vi "Drive_Teleop.vi"(1 "Joystick_Out":T1={"Pilot Left Joystick X"=0.007874015748031496, "Pilot Left Joystick Y"=-0.0, "Pilot A Button"=FALSE, "Pilot B Button"=FALSE, "Pilot X Button"=FALSE, "Pilot Y Button"=FALSE, "Pilot Left Bumper"=FALSE, "Pilot Right Bumper"=FALSE, "Pilot View Button"=FALSE, "Pilot Menu Button"=FALSE, "Pilot Left Joystick Press"=FALSE, "Pilot Right Joystick Press"=FALSE, "Pilot Left Trigger"=0.0, "Pilot Right Joystick X"=0.0, "Pilot Right Joystick Y"=0.0, "Pilot Right Trigger"=0.0, "Copilot Left Joystick X"=0.05511811023622047, "Copilot Left Joystick Y"=0.023622047244094488, "Copilot A Button"=FALSE, "Copilot B Button"=FALSE, "Copilot X Button"=FALSE, "Copilot Y Button"=FALSE, "Copilot Left Bumper"=FALSE, "Copilot Right Bumper"=FALSE, "Copilot View Button"=FALSE, "Copilot Menu Button"=FALSE, "Copilot Left Joystick Press"=FALSE, "Copilot Right Joystick Press"=FALSE, "Copilot Left Trigger"=0.0, "Copilot Right Joystick X"=-0.015748031496062992, "Copilot Right Joystick Y"=0.05511811023622047, "Copilot Right Trigger"=0.0, "Pilot D-pad North"=FALSE, "Pilot D-pad South"=FALSE, "Pilot D-pad East"=FALSE, "Pilot D-pad West"=FALSE, "Pilot D-pad NE "=FALSE, "Pilot D-pad SE"=FALSE, "Pilot D-pad SW"=FALSE, "Pilot D-pad NW"=FALSE, "CoPilot D-pad North"=FALSE, "CoPilot D-pad South"=FALSE, "CoPilot D-pad East"=FALSE, "CoPilot D-pad West"=FALSE, "CoPilot D-pad NE"=FALSE, "CoPilot D-pad SE"=FALSE, "CoPilot D-pad SW"=FALSE, "CoPilot D-pad NW"=FALSE, "Pilot Left Trigger Pressed"=FALSE, "Pilot Right Trigger Pressed"=FALSE, "CoPilot Left Trigger Pressed"=FALSE, "CoPilot Right Trigger Pressed"=FALSE}) -> ()   [LabVIEW 2020]
uses:
  Utility VIs/Joystick_Controls.ctl
  Subsystems/Drive/Drive_Cluster.ctl
  Subsystems/Drive/Drive_Control_States.ctl
  Subsystems/Drive/Drive_Orientation_States.ctl
  <vilib>/Rock Robotics/WPI/DriverStation/WPI_DriverStationRobotMode2.ctl
  Globals/Drive_Globals.vi
  Robot Global Data.vi
  Systems/Shooter/Determiner/Shooter_Globals.vi
  <vilib>/Analysis/NI_AALBase.lvlib
  <vilib>/Analysis/baseanly.llb/Unit Vector (DBL).vi
panel:
  in  "SWM_Magnitude_Limit":dbl=0.3
  in  "Slew Rate Limit (/s)":dbl=1.0
  in  "sizeOfAverageArray":i32=3
  in  "Rotation Maximum":dbl(slide)=0.5 min=0.3 max=1.0 scale=0.3..1.0
  in  "Rotation Scaling":dbl(slide)=2.0 min=1.0 max=4.0 scale=1.0..4.0
  in  "Rotation Deadband":dbl(slide)=0.1 min=0.0 max=0.25 scale=0.0..0.25
  in  "Strafe Maximum":dbl(slide)=1.0 min=0.3 max=1.0 scale=0.3..1.0
  in  "Strafe Scaling":dbl(slide)=1.0 min=1.0 max=4.0 scale=1.0..4.0
  in  "Strafe Deadband":dbl(slide)=0.1 min=0.0 max=0.25 scale=0.0..0.25
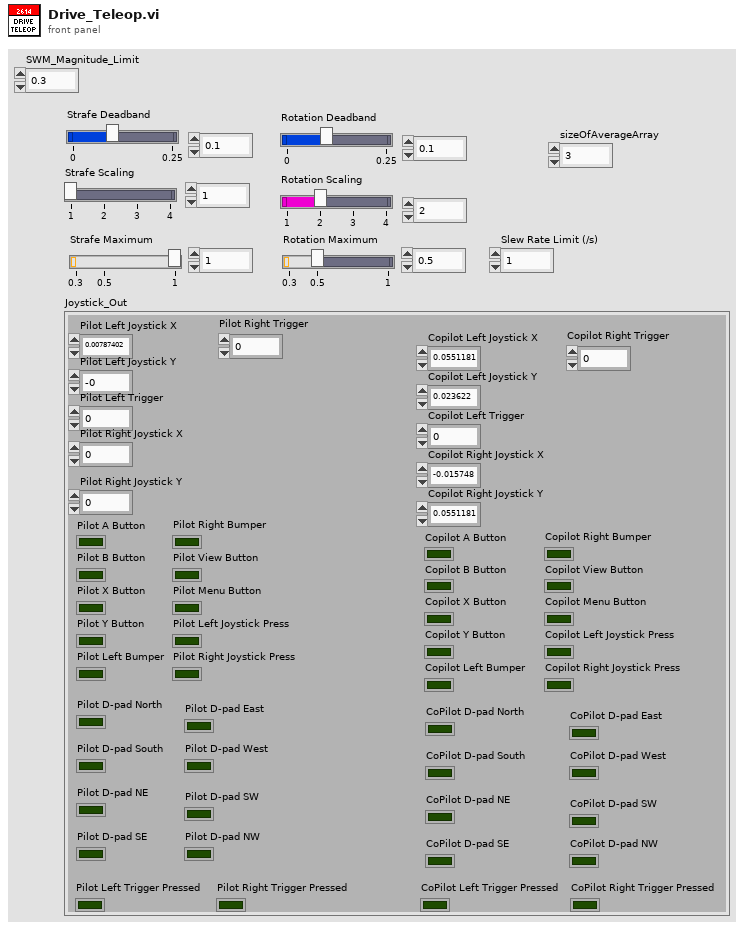
[diagram p1: front panel]
types:
  T1 = typedef "Joystick_Controls.ctl" = cluster{"Pilot Left Joystick X":dbl, "Pilot Left Joystick Y":dbl, "Pilot A Button":bool, "Pilot B Button":bool, "Pilot X Button":bool, "Pilot Y Button":bool, "Pilot Left Bumper":bool, "Pilot Right Bumper":bool, "Pilot View Button":bool, "Pilot Menu Button":bool, "Pilot Left Joystick Press":bool, "Pilot Right Joystick Press":bool, "Pilot Left Trigger":dbl, "Pilot Right Joystick X":dbl, "Pilot Right Joystick Y":dbl, "Pilot Right Trigger":dbl, "Copilot Left Joystick X":dbl, "Copilot Left Joystick Y":dbl, "Copilot A Button":bool, "Copilot B Button":bool, "Copilot X Button":bool, "Copilot Y Button":bool, "Copilot Left Bumper":bool, "Copilot Right Bumper":bool, "Copilot View Button":bool, "Copilot Menu Button":bool, "Copilot Left Joystick Press":bool, "Copilot Right Joystick Press":bool, "Copilot Left Trigger":dbl, "Copilot Right Joystick X":dbl, "Copilot Right Joystick Y":dbl, "Copilot Right Trigger":dbl, "Pilot D-pad North":bool, "Pilot D-pad South":bool, "Pilot D-pad East":bool, "Pilot D-pad West":bool, "Pilot D-pad NE ":bool, "Pilot D-pad SE":bool, "Pilot D-pad SW":bool, "Pilot D-pad NW":bool, "CoPilot D-pad North":bool, "CoPilot D-pad South":bool, "CoPilot D-pad East":bool, "CoPilot D-pad West":bool, "CoPilot D-pad NE":bool, "CoPilot D-pad SE":bool, "CoPilot D-pad SW":bool, "CoPilot D-pad NW":bool, "Pilot Left Trigger Pressed":bool, "Pilot Right Trigger Pressed":bool, "CoPilot Left Trigger Pressed":bool, "CoPilot Right Trigger Pressed":bool}
  T2 = typedef "Drive_Orientation_States.ctl" = enum16{"Robot-Oriented", "Field-Oriented"}
  T3 = typedef "WPI_DriverStationRobotMode2.ctl" = enum16{"Autonomous Disabled", "Autonomous Enabled", "Teleop Disabled", "Teleop Enabled", "Disconnected", "Finish", "Test Disabled", "Test Enabled", "Emergency Stopped"}
  T4 = typedef "Drive_Cluster.ctl" = cluster{"Control_State":T5, "Vertical_Throttle":dbl, "Lateral_Throttle":dbl, "Rotational_Throttle":dbl, "Strafe_In_Deadband":bool, "Rotation_In_Deadband":bool, "Orientation_State":T2, "Parameters":dbl[], "Step":i32, "Auto_Notifier":refnum<notifier>, "PathName":string, "Raw_X":dbl, "Raw_Y":dbl, "Pivot_Driving?":bool}
  T5 = typedef "Drive_Control_States.ctl" = enum16{"No-Op", "Manual_Control", "Command_DriveDistanceAtAngle", "Command_DrivePath", "Command_SetRobotPose", "Command_Rotate"}
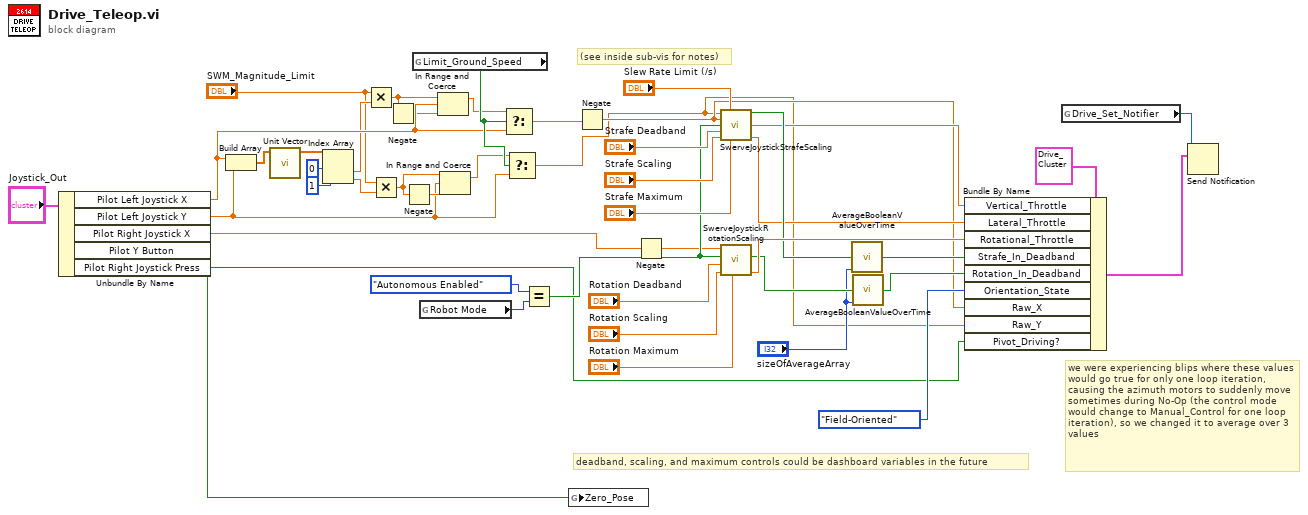
[diagram p0: block diagram]
diagram:
  # "we were experiencing blips where these values would go true for only one loop iteration, causing the azimuth motors to suddenly move sometimes during No-Op (the control mode would change to Manual_Control for one loop iteration), so we changed it to average over 3 values"
  # "(see inside sub-vis for notes)"
  # "deadband, scaling, and maximum controls could be dashboard variables in the future"
  n1 = Unbundle By Name("Joystick_Out") -> ("Pilot Left Joystick X"=w10:dbl, "Pilot Left Joystick Y"=w2:dbl, "Pilot Right Joystick X"=w42:dbl, "Pilot Y Button"=w26:bool, "Pilot Right Joystick Press"=w19:bool)
  n2 = Build Array(w10, w2) -> (w15:dbl[])
  n3 = call-poly <vilib>:"Unit Vector.vi"("Input Vector"=w15) -> ("Unit Vector"=w14:dbl[])  [unwired: 8 in, 2 out]
  n4 = Index Array(array=w14, index #1=0 ("index"), index #2=1 ("index")) -> (element #1=w9:dbl, element #2=w5:dbl)
  n5 = Multiply(x="SWM_Magnitude_Limit", y=w9) -> (x*y=w8:dbl)
  n6 = Multiply(x="SWM_Magnitude_Limit", y=w5) -> (x*y=w3:dbl)
  n7 = Negate(x=w8) -> (-x=w7:dbl)
  n8 = Negate(x=w3) -> (-x=w4:dbl)
  n9 = global read "Shooter_Globals.vi" "Limit_Ground_Speed"() -> (w16:bool)
  n10 = global read "Robot Global Data.vi" "Robot Mode"() -> (w34:T3)
  n11 = In Range and Coerce(upper limit=w8, x=w10, lower limit=w7) -> (coerced(x)=w11:dbl)  [unwired: 1 out]
  n12 = In Range and Coerce(upper limit=w3, x=w2, lower limit=w4) -> (coerced(x)=w1:dbl)  [unwired: 1 out]
  n13 = Select(t=w11, s=w16, f=w10) -> (s? t:f=w18:dbl)
  n14 = Select(t=w1, s=w16, f=w2) -> (s? t:f=w17:dbl)
  n15 = Equal?(x=WPI_DriverStationRobotMode2."Autonomous Enabled" ("Robot Mode"), y=w34) -> (x = y?=w33:bool)
  n16 = global write "Drive_Globals.vi" "Zero_Pose"(w26) -> ()
  n17 = Negate(x=w18) -> (-x=w20:dbl)
  n18 = Negate(x=w42) -> (-x=w25:dbl)
  n19 = call "SwerveJoystickStrafeScaling.vi"("Raw Joystick X"=w17, "Slew Rate Limit (/s)"="Slew Rate Limit (/s)", "Raw Joystick Y"=w20, "Auto Control"=w33, "Strafe Deadband"="Strafe Deadband", "Strafe Scaling"="Strafe Scaling", "Strafe Maximum"="Strafe Maximum") -> ("In Deadband"=w31:bool, "Scaled Joystick X"=w22:dbl, "Scaled Joystick Y"=w21:dbl)  [unwired: 6 in]
  n20 = call "SwerveJoystickRotationScaling.vi"("Rotation Maximum"="Rotation Maximum", "Rotation Scaling"="Rotation Scaling", "Rotation Deadband"="Rotation Deadband", "Auto Control"=w33, "Raw Joystick Rotation"=w25) -> ("Scaled Joystick Rotation"=w32:dbl, "In Deadband"=w29:bool)  [unwired: 4 in]
  n21 = call "AverageBooleanValueOverTime.vi"("input boolean"=w31, "sizeOfAverageArray (5)"="sizeOfAverageArray") -> ("averaged"=w30:bool)  [unwired: 13 in]
  n22 = call "AverageBooleanValueOverTime.vi"("input boolean"=w29, "sizeOfAverageArray (5)"="sizeOfAverageArray") -> ("averaged"=w28:bool)  [unwired: 13 in]
  n23 = Bundle By Name(cluster=T4 {"Control_State"=enum."Manual_Control", "Vertical_Throttle"=0.0, "Lateral_Throttle"=0.0, "Rotational_Throttle"=0.0, "Strafe_In_Deadband"=FALSE, "Rotation_In_Deadband"=FALSE, "Orientation_State"=enum."Robot-Oriented", "Parameters"=[], "Step"=0, "Auto_Notifier"=refnum, "PathName"="", "Raw_X"=0.0, "Raw_Y"=0.0, "Pivot_Driving?"=FALSE} ("notification"), "Vertical_Throttle"=w22, "Lateral_Throttle"=w21, "Rotational_Throttle"=w32, "Strafe_In_Deadband"=w30, "Rotation_In_Deadband"=w28, "Orientation_State"=Drive_Orientation_States."Field-Oriented", "Raw_X"=w20, "Raw_Y"=w17, "Pivot_Driving?"=w19) -> (w46:T4)
  n24 = global read "Drive_Globals.vi" "Drive_Set_Notifier"() -> (w43:refnum<notifier>)
  n25 = Send Notification(notification=w46, notifier=w43) -> ()  [unwired: 1 in, 2 out]
